vi "Tree Data Types and XML Example.vi"() -> ()   [LabVIEW 2017, in "Tree API.lvlib" / "Tree.lvclass"]
uses:
  Tree.lvclass
  API/Set Meta Data.vi
  API/List Roots.vi
  API/Set Attributes Tree Data.vi
panel:
  out "XML String":string="<Parent MetaData=\"You can add descriptions to your trees.\">\n\n<Child>\n<MyInteger Type=\"Int\">\r\n12\r\n</MyInteger>\r\n<My1DInteger Type=\"1D Int\">\r\n23, 34\r\n</My1DInteger>\r\n<My2DInteger Type=\"2D Int\">\r\n23, 34;\r\n45, 56\r\n</My2DInteger>\r\n<MyPath Type=\"Path\">\r\n\"test.llb\"\r\n</MyPath>\r\n<My1DPath Type=\"1D Path\">\r\n\"test.llb\", \"\\\\\\\\netpath\\\\\"\r\n</My1DPath>\r\n<My2DPath Type=\"2D Path\">\r\n\"test.llb\", \"\\\\\\\\netpath\\\\\";\r\n\"a\", \"b\"\r\n</My2DPath>\r\n<MyBool Type=\"Bool\">\r\nTRUE\r\n</MyBool>\r\n<My1DBool Type=\"1D Bool\">\r\nTRUE, FALSE\r\n</My1DBool>\r\n<My2DBoolArray Type=\"2D Bool\">\r\nFALSE, TRUE;\r\nFALSE, TRUE\r\n</My2DBoolArray>\r\n<MyFloat Type=\"Flt\">\r\n3.14\r\n</MyFloat>\r\n<My1DFloat Type=\"1D Flt\">\r\n9.8596, 97.211712\r\n</My1DFloat>\r\n<My2DFloat Type=\"2D Flt\">\r\n9.8596, 97.211712;\r\n97.211712, 9450.116981\r\n</My2DFloat>\r\n<My_String Type=\"String\" MetaData=\"Any Tree Data class can use this field.\">\r\n\"Foo\"\r\n</My_String>\r\n<My_1D_String Type=\"1D String\">\r\n\"d\"\r\n</My_1D_String>\r\n<My_2D_String Type=\"2D String\">\r\n\"Foo\", \"Bar\\\\\";\r\n\"Bar\", \"&lt;&gt;&apos;&quot;&amp;\\;\\,\\\\\"\r\n</My_2D_String>\n\n</Child>\n</Parent>"
  in  "Tree":string(tree)
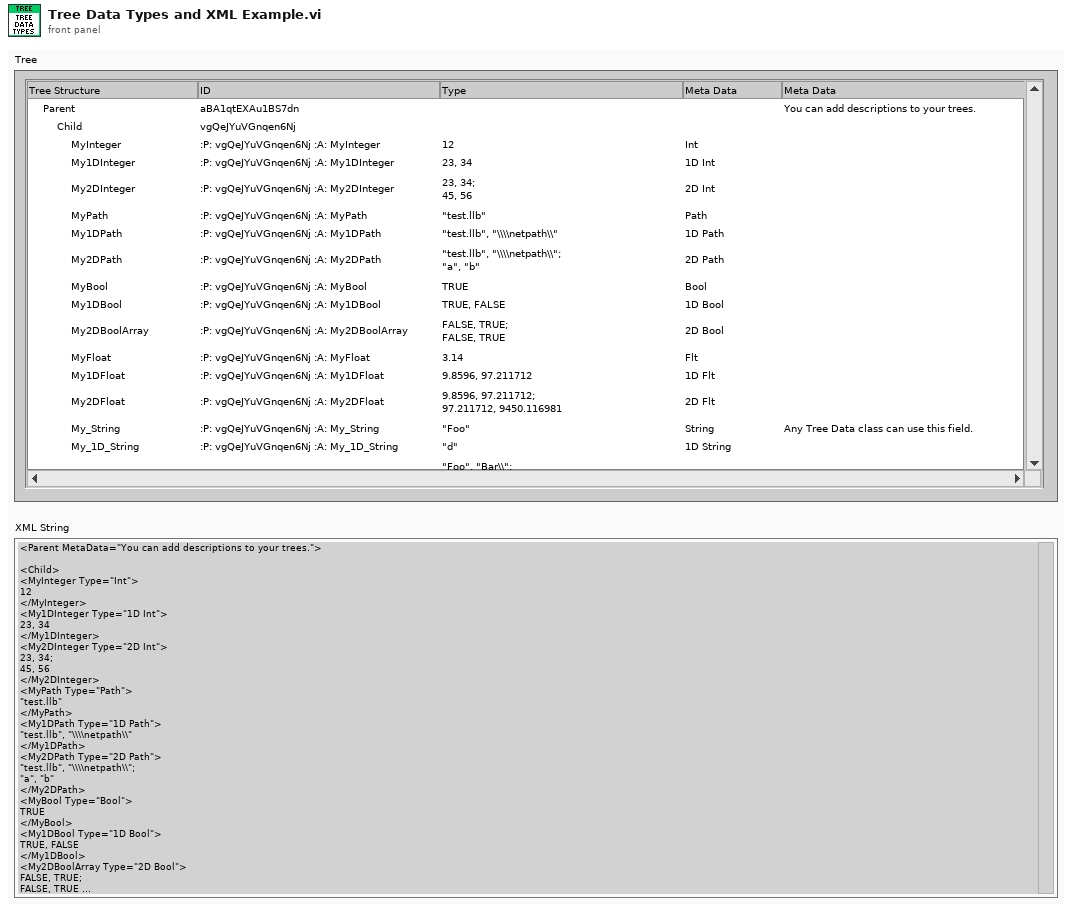
[diagram p1: front panel]
types:
  T1 = cluster{"Left Cell String":string, "Child Text":string[], "Child Tag":string, "Item Indent":i32, "Child Only?":bool, "Glyph Index":i32}[]
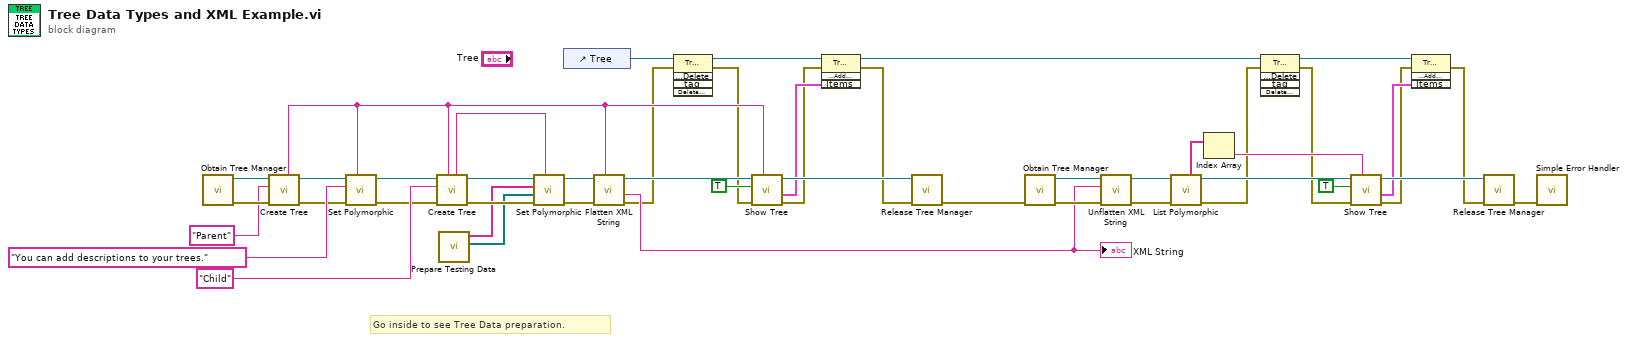
[diagram p0: block diagram]
diagram:
  # "Go inside to see Tree Data preparation."
  n1 = call "Obtain Tree Manager.vi"() -> ("Error Out"=w45:errorcluster, "Tree"=w46:refnum<data-value>)  [unwired: 10 in]
  n2 = call "Create Tree.vi"("Error In"=w45, "Name"="Parent", "Tree Manager"=w46) -> ("Error Out"=w17:errorcluster, "Tree Manager"=w18:refnum<data-value>, "Unique ID"=w19:string)  [unwired: 6 in]
  n3 = call-poly "Set Polymorphic.vi"("Tree ID"=w19, "Error In"=w17, "Meta Data"="You can add descriptions to your trees.", "Tree Manager"=w18) -> ("Error Out"=w28:errorcluster, "Tree Manager"=w29:refnum<data-value>)  [unwired: 6 in]
  n4 = call "Create Tree.vi"("Parent ID (empty)"=w19, "Error In"=w28, "Name"="Child", "Tree Manager"=w29) -> ("Error Out"=w42:errorcluster, "Tree Manager"=w43:refnum<data-value>, "Unique ID"=w25:string)  [unwired: 5 in]
  n5 = call "Prepare Testing Data.vi"() -> ("Attr Data"=w31:refnum<class "Tree Data.lvclass">[], "Attr Names"=w30:string[])  [unwired: 10 in]
  n6 = call-poly "Set Polymorphic.vi"("Tree ID"=w25, "Error In"=w42, "Attributes Values"=w31, "Attributes Names"=w30, "Tree Manager"=w43) -> ("Error Out"=w24:errorcluster, "Tree Manager"=w26:refnum<data-value>)  [unwired: 4 in, 1 out]
  n7 = control-ref of="Tree"() -> (w13:refnum<vi>)
  n8 = call "Flatten XML String.vi"("Root ID"=w19, "Error In"=w24, "Tree"=w26) -> ("Error Out"=w8:errorcluster, "XML String"=w35:string, "Tree"=w34:refnum<data-value>)  [unwired: 6 in]
  "XML String" <- w35
  n9 = invoke class="Tree (strict)" method="Edit Tree Items.Delete"(reference=w13, error in=w8) -> (reference out=w14:refnum<vi>, error out=w7:errorcluster)  [unwired: 3 in, 3 out]
  n10 = call "Show Tree.vi"("Root ID"=w19, "Error In"=w7, "Show IDs (False)"=TRUE, "Tree"=w34) -> ("Error Out"=w4:errorcluster, "Items Out"=w12:T1, "Tree"=w33:refnum<data-value>)  [unwired: 5 in]
  n11 = invoke class="Tree (strict)" method="Edit Tree Items.Add Multiple Items to End"(reference=w14, error in=w4, "Items"=w12) -> (reference out=w10:refnum<vi>, error out=w3:errorcluster)  [unwired: 1 in, 2 out]
  n12 = call "Release Tree Manager.vi"("Error In"=w3, "Tree"=w33) -> ("Error Out"=w23:errorcluster)  [unwired: 9 in]
  n13 = call "Obtain Tree Manager.vi"("Error In"=w23) -> ("Error Out"=w39:errorcluster, "Tree"=w40:refnum<data-value>)  [unwired: 9 in]
  n14 = call "Unflatten XML String.vi"("Error In"=w39, "XML String"=w35, "Tree"=w40) -> ("Error Out"=w37:errorcluster, "Tree"=w38:refnum<data-value>)  [unwired: 7 in]
  n15 = call-poly "List Polymorphic.vi"("Error In"=w37, "Tree"=w38) -> ("Error Out"=w6:errorcluster, "Tree"=w36:refnum<data-value>, "Roots IDs"=w32:string[])  [unwired: 6 in, 1 out]
  n16 = Index Array(array=w32) -> (element=w21:string)  [unwired: 1 in]
  n17 = invoke class="Tree (strict)" method="Edit Tree Items.Delete"(reference=w10, error in=w6) -> (reference out=w11:refnum<vi>, error out=w5:errorcluster)  [unwired: 3 in, 3 out]
  n18 = call "Show Tree.vi"("Root ID"=w21, "Error In"=w5, "Show IDs (False)"=TRUE, "Tree"=w36) -> ("Error Out"=w2:errorcluster, "Items Out"=w9:T1, "Tree"=w22:refnum<data-value>)  [unwired: 5 in]
  n19 = invoke class="Tree (strict)" method="Edit Tree Items.Add Multiple Items to End"(reference=w11, error in=w2, "Items"=w9) -> (error out=w1:errorcluster)  [unwired: 1 in, 3 out]
  n20 = call "Release Tree Manager.vi"("Error In"=w1, "Tree"=w22) -> ("Error Out"=w41:errorcluster)  [unwired: 9 in]
  n21 = call <vilib>:"Simple Error Handler.vi"("error in (no error)"=w41) -> ()  [unwired: 4 in, 5 out]
